vi "Timeout.vi"(8 "error in (no error)":errorcluster, 10 "Context in":refnum<class "Context.lvclass">, 11 "Active in":refnum<class "Active.lvclass">) -> (0 "error out":errorcluster, 2 "Context out":refnum<class "Context.lvclass">, 3 "State out":refnum<class "State.lvclass">)   [LabVIEW 2024, in "State.lvlib" / "Active.lvclass"]
uses:
  Active.lvclass
  C:/Users/uspoaotto/OneDrive - Oregon Tool/Desktop/working copies/stateMachineActor/src/State Machine/State/Container State/Container State.lvclass
  State/State.lvclass
  Context/Context/Context.lvclass
  Active.lvclass/Active.ctl
  Timed Out/Timed Out.lvclass
  C:/Users/uspoaotto/OneDrive - Oregon Tool/Desktop/working copies/stateMachineActor/src/State Machine/State/State/State.lvclass
  C:/Users/uspoaotto/OneDrive - Oregon Tool/Desktop/working copies/stateMachineActor/src/State Machine/State/Active/Active.lvclass
  C:/Users/uspoaotto/OneDrive - Oregon Tool/Desktop/working copies/stateMachineActor/src/State Machine/State/Timed Out/Timed Out.lvclass
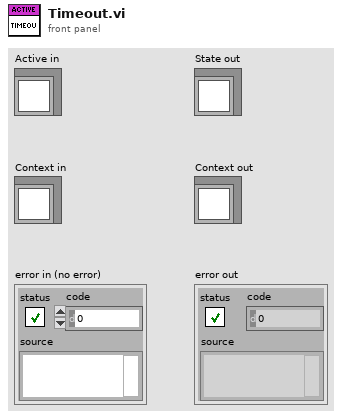
[diagram p1: front panel]
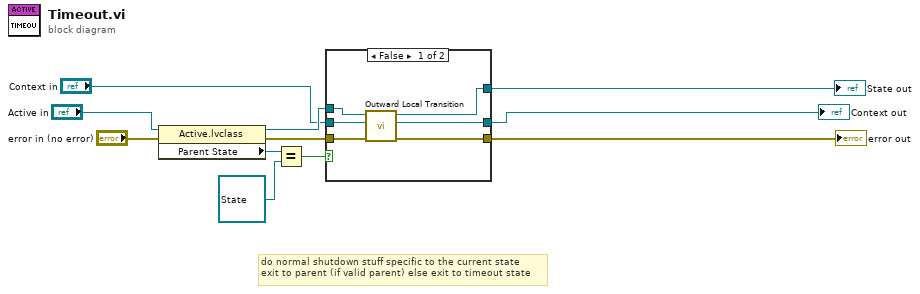
[diagram p0: block diagram]
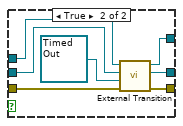
[diagram p2: hidden frame]
diagram:
  # "do normal shutdown stuff specific to the current state\nexit to parent (if valid parent) else exit to timeout state"
  n1 = property class="Active.lvclass"(reference="Active in", error in="error in (no error)") -> (reference out=w7:refnum<class "Active.lvclass">, error out=w2:errorcluster, "Parent State"=w1:refnum<class "State.lvclass">)
  n2 = Equal?(x=w1, y=refnum<class "State.lvclass"> refnum ("State.lvlib:State.lvclass")) -> (x = y?=w8:bool)
  n3 = case shown="False" w8 {
    tunnel: w7 -> [w17 w24]
    tunnel: "Context in" -> [w16 w22]
    tunnel: [w13 w21] -> w5
    tunnel: [w15 w20] -> w4
    tunnel: [w14 w19] -> w3
    tunnel: w2 -> [w12 w18]
    frame False {
      n4 = call "Outward Local Transition.vi"("error in (no error)"=w12, "Context in"=w16, "State in"=w17) -> ("error out"=w14:errorcluster, "Context out"=w15:refnum<class "Context.lvclass">, "State out"=w13:refnum<class "State.lvclass">)  [unwired: 6 in]
    }
    frame True {
      n5 = call "External Transition.vi"("error in (no error)"=w18, "Target State"=refnum<class "Timed Out.lvclass"> refnum ("State.lvlib:Timed Out.lvclass"), "Context in"=w22, "State in"=w24) -> ("error out"=w19:errorcluster, "Context out"=w20:refnum<class "Context.lvclass">, "State out"=w21:refnum<class "State.lvclass">)  [unwired: 5 in]
    }
  }
  "error out" <- w3
  "State out" <- w5
  "Context out" <- w4
